vi "Get Class Path by Name.vi"(8 "Error in":errorcluster caption="Error in (no error)", 10 "Original ClassInfo":T1, 11 "String":string) -> (0 "Error out":errorcluster, 2 "output cluster":T1)   [LabVIEW 2016, in "LV Object Event Registration Node.xnode"]
uses:
  LV Object Event Registration Node.xnode
  LOER_ClassInfo.ctl
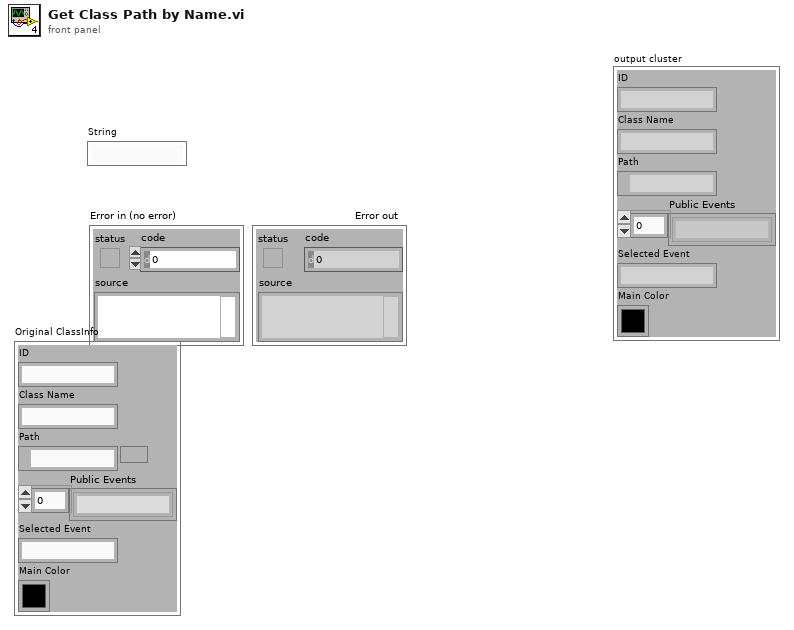
[diagram p1: front panel]
types:
  T1 = typedef "LV Object Event Registration Node.xnode/LOER_ClassInfo.ctl" = cluster{"ID":string, "Class Name":string, "Path":path, "Public Events":string[], "Selected Event":string, "Main Color":u32}
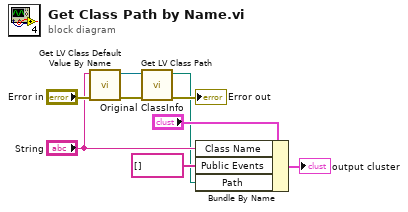
[diagram p0: block diagram]
diagram:
  n1 = call <vilib>:"Get LV Class Default Value By Name.vi"("error in (no error)"="Error in", "class name"="String") -> ("error out"=w9:errorcluster, "object"=w7:refnum<class>)  [unwired: 8 in]
  n2 = call <vilib>:"Get LV Class Path.vi"("error in (no error)"=w9, "object"=w7) -> ("error out"=→"Error out":errorcluster, "class path"=w1:path)  [unwired: 8 in]
  n3 = Bundle By Name(cluster="Original ClassInfo", "Class Name"="String", "Public Events"=string[] [], "Path"=w1) -> (→"output cluster":T1)
